vi "PumpDemo.vi"() -> ()   [LabVIEW 2009]
doc: "Demos the pump active object.\n\nwww.sciware.com.au"
uses:
  SimPump/SimPump.lvclass
panel:
  in  "Flow Rate B":dbl=2.0 caption="Flow Rate"
  out "Volume Pumped B":dbl caption="Volume Pumped"
  out "State B":bool caption="State"
  in  "Volume to Pump B":dbl=3.0 caption="Volume to Pump"
  in  "pump vol B":bool
  in  "off B":bool
  in  "on B":bool
  in  "Flow Rate A":dbl=1.0 caption="Flow Rate"
  out "Volume Pumped A":dbl caption="Volume Pumped"
  out "State A":bool caption="State"
  in  "Volume to Pump A":dbl=5.0 caption="Volume to Pump"
  in  "pump vol A":bool
  in  "off A":bool
  in  "on A":bool
  in  "stop":bool
  # "PUMP B"
  # "PUMP A"
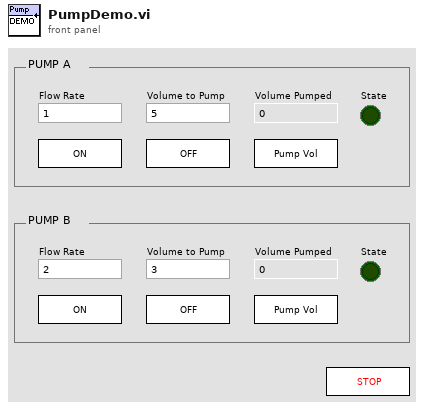
[diagram p1: front panel]
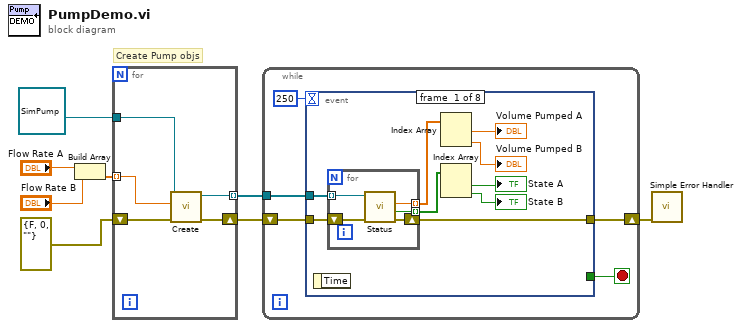
[diagram p0: block diagram]
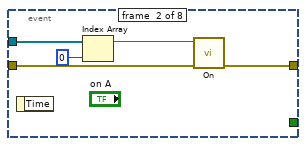
[diagram p2: hidden frame]
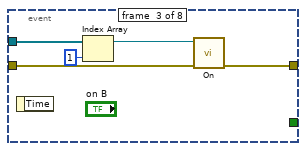
[diagram p3: hidden frame]
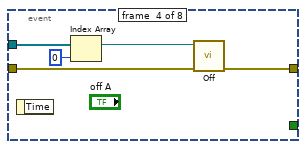
[diagram p4: hidden frame]
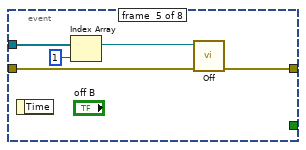
[diagram p5: hidden frame]
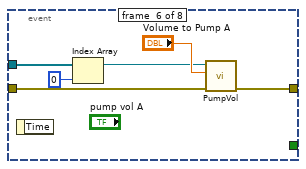
[diagram p6: hidden frame]
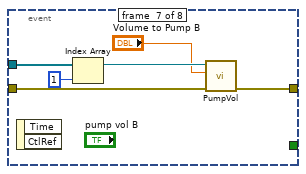
[diagram p7: hidden frame]
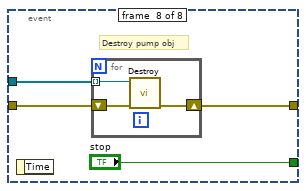
[diagram p8: hidden frame]
diagram:
  # "Create Pump objs"
  n1 = Build Array("Flow Rate A", "Flow Rate B") -> (w5:dbl[])
  n2 = for {
    tunnel: refnum<class "SimPump.lvclass"> refnum ("obj") -> [w13]
    tunnel: [w9] -> w8 mode=indexing
    tunnel: w5 -> [w12] mode=indexing
    shift-right: [w10] -> w3
    shift-left: errorcluster {"status"=FALSE, "code"=0, "source"=""} ("error out") -> [w11]
    n3 = call-dynamic "Create.vi"("error in (no error)"=w11, "flow rate"=w12, "obj"=w13) -> ("error out"=w10:errorcluster, "obj out"=w9:refnum<class "SimPump.lvclass">)  [unwired: 7 in]
  }
  n4 = while {
    tunnel: w8 -> [w17]
    shift-right: [w15] -> w2
    shift-left: w3 -> [w16]
    stop <- w14 stop-if-true
    n5 = event shown="[7] \"stop\": Value Change" {
      selector: _ -> [_ _ _ _ _ _ _ _]
      dyn-events: _ -> [_ _ _ _ _ _ _ _]
      timeout: 250 -> [_ _ _ _ _ _ _ _]
      tunnel: w17 -> [w25 w35 w40 w45 w50 w55 w62 w65]
      tunnel: w16 -> [w27 w37 w42 w47 w52 w58 w64 w68]
      tunnel: [w26 w36 w41 w46 w51 w57 w63 w67] -> w15
      tunnel: [_ _ _ _ _ _ _ "stop"] -> w14
      event #0 {
        n6 = event-data() -> ()  [unwired: 1 in, 1 out]
        n7 = for {
          tunnel: [w30] -> w21 mode=indexing
          tunnel: [w29] -> w24 mode=indexing
          tunnel: w25 -> [w28] mode=indexing
          shift-right: [w31] -> w26
          shift-left: w27 -> [w32]
          n8 = call-dynamic "Status.vi"("error in (no error)"=w32, "SimPump in"=w28) -> ("error out"=w31:errorcluster, "state"=w30:bool, "volume pumped"=w29:dbl)  [unwired: 6 in, 1 out]
        }
        n9 = Index Array(array=w24) -> (element #1=→"Volume Pumped A":dbl, element #2=→"Volume Pumped B":dbl)  [unwired: 2 in]
        n10 = Index Array(array=w21) -> (element #1=→"State A":bool, element #2=→"State B":bool)  [unwired: 2 in]
      }
      event #1 {
        n11 = event-data() -> ()  [unwired: 1 in, 1 out]
        n12 = Index Array(array=w35, index=0) -> (element=w33:refnum<class "SimPump.lvclass">)
        n13 = call-dynamic "On.vi"("error in (no error)"=w37, "SimPump in"=w33) -> ("error out"=w36:errorcluster)  [unwired: 8 in, 1 out]
      }
      event #2 {
        n14 = event-data() -> ()  [unwired: 1 in, 1 out]
        n15 = Index Array(array=w40, index=1) -> (element=w38:refnum<class "SimPump.lvclass">)
        n16 = call-dynamic "On.vi"("error in (no error)"=w42, "SimPump in"=w38) -> ("error out"=w41:errorcluster)  [unwired: 8 in, 1 out]
      }
      event #3 {
        n17 = event-data() -> ()  [unwired: 1 in, 1 out]
        n18 = Index Array(array=w45, index=0) -> (element=w44:refnum<class "SimPump.lvclass">)
        n19 = call-dynamic "Off.vi"("error in (no error)"=w47, "SimPump in"=w44) -> ("error out"=w46:errorcluster)  [unwired: 8 in, 1 out]
      }
      event #4 {
        n20 = event-data() -> ()  [unwired: 1 in, 1 out]
        n21 = Index Array(array=w50, index=1) -> (element=w49:refnum<class "SimPump.lvclass">)
        n22 = call-dynamic "Off.vi"("error in (no error)"=w52, "SimPump in"=w49) -> ("error out"=w51:errorcluster)  [unwired: 8 in, 1 out]
      }
      event #5 {
        n23 = event-data() -> ()  [unwired: 1 in, 1 out]
        n24 = Index Array(array=w55, index=0) -> (element=w54:refnum<class "SimPump.lvclass">)
        n25 = call-dynamic "PumpVol.vi"("error in (no error)"=w58, "volume to pump"="Volume to Pump A", "SimPump in"=w54) -> ("error out"=w57:errorcluster)  [unwired: 7 in, 1 out]
      }
      event #6 {
        n26 = event-data() -> ()  [unwired: 1 in, 2 out]
        n27 = Index Array(array=w62, index=1) -> (element=w61:refnum<class "SimPump.lvclass">)
        n28 = call-dynamic "PumpVol.vi"("error in (no error)"=w64, "volume to pump"="Volume to Pump B", "SimPump in"=w61) -> ("error out"=w63:errorcluster)  [unwired: 7 in, 1 out]
      }
      event #7 {
        # "Destroy pump obj"
        n29 = event-data() -> ()  [unwired: 1 in, 1 out]
        n30 = for {
          shift-right: [w70] -> w67
          shift-left: w68 -> [w71]
          tunnel: w65 -> [w69] mode=indexing
          n31 = call-dynamic "Destroy.vi"("error in (no error)"=w71, "obj"=w69) -> ("error out"=w70:errorcluster)  [unwired: 9 in]
        }
      }
    }
  }
  n32 = call <vilib>:"Simple Error Handler.vi"("error in (no error)"=w2) -> ()  [unwired: 4 in, 5 out]
